vi "ExampleClient.vi"() -> ()   [LabVIEW 2013]
panel:
  out "Response":string
  out "Command":string
  in  "VarSet":T1(array[cluster])
  in  "Send Seq":bool
  in  "Send Now":bool
  in  "Send Mulligan":bool
  in  "Mulligan FileNum":i32
  in  "stop":bool
  in  "IP Address":string="127.0.0.1"
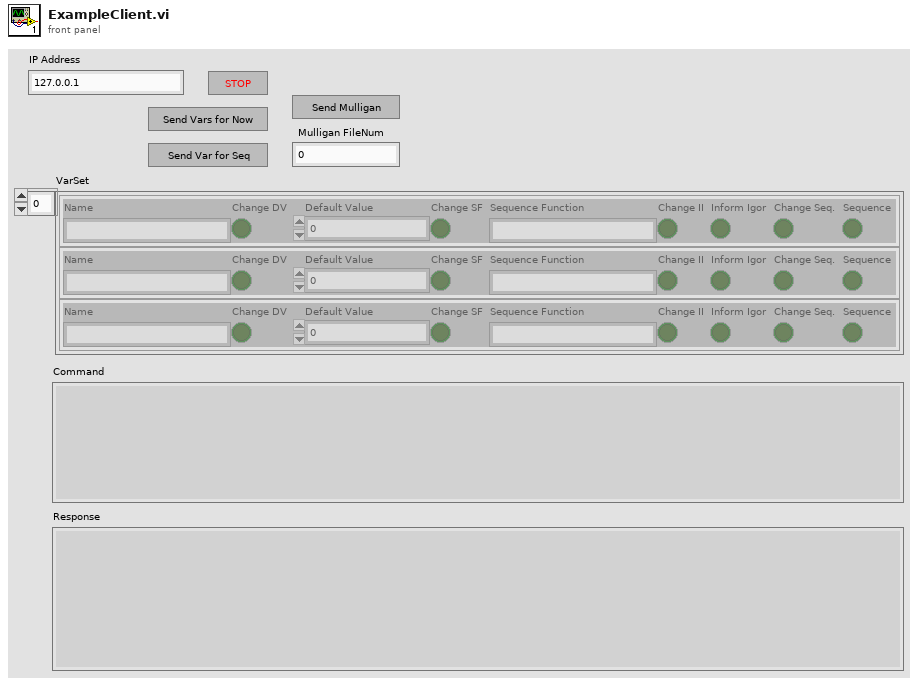
[diagram p1: front panel]
types:
  T1 = cluster{"Name":string, "Change DV":bool, "Default Value":dbl, "Change SF":bool, "Sequence Function":string, "Change II":bool, "Inform Igor":bool, "Change Seq.":bool, "Sequence":bool}[]
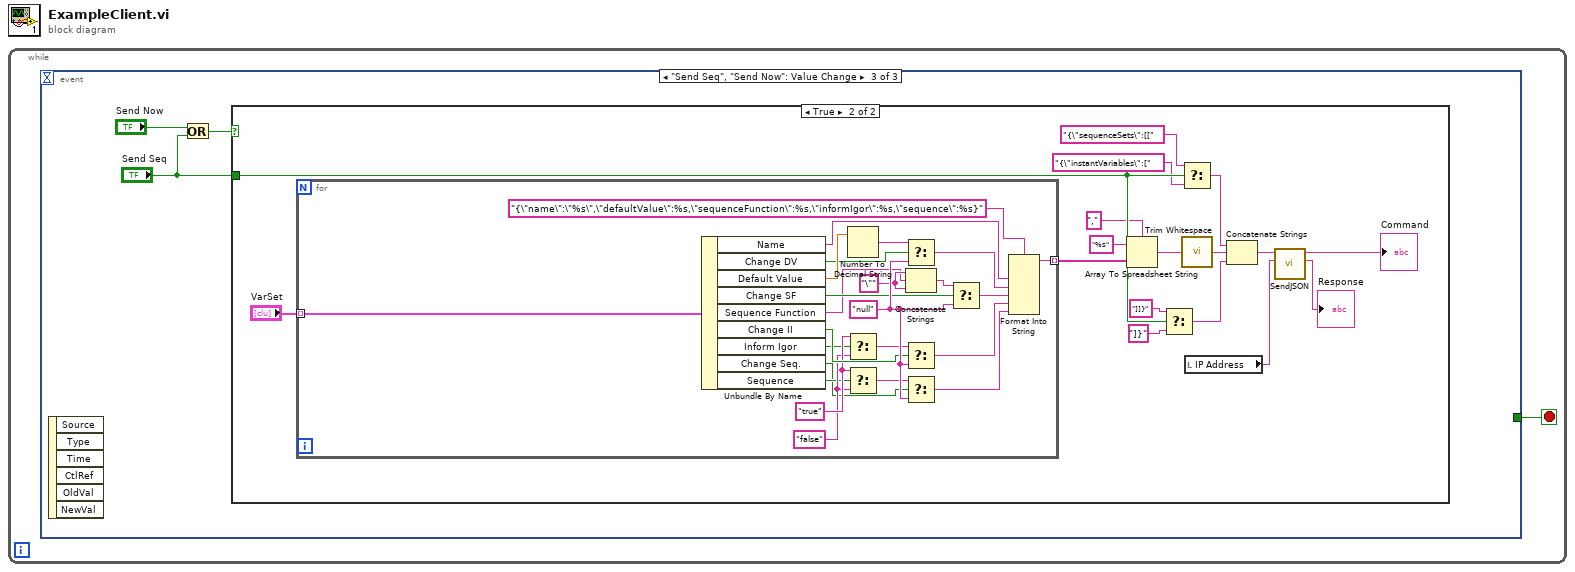
[diagram p0: block diagram]
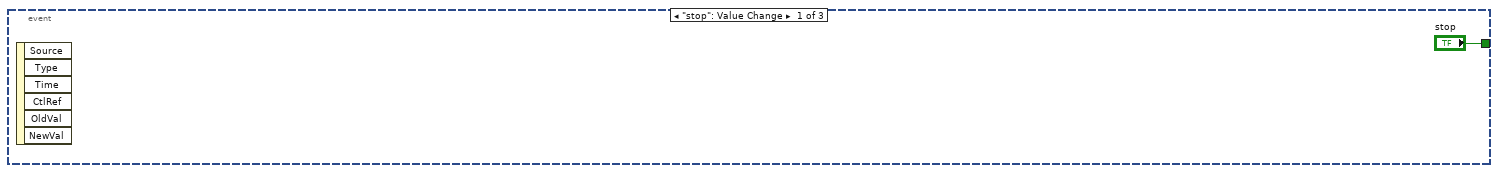
[diagram p2: hidden frame]
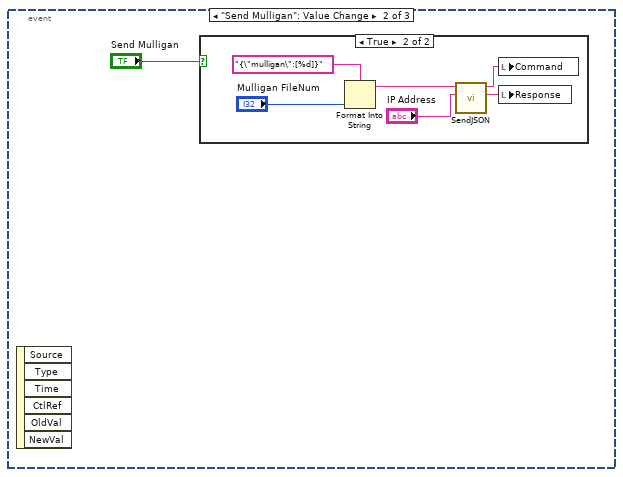
[diagram p3: hidden frame]
diagram:
  n1 = while {
    stop <- w1 stop-if-true
    n2 = event shown="[2] \"Send Seq\", \"Send Now\": Value Change" {
      selector: _ -> [_ _ _]
      dyn-events: _ -> [_ _ _]
      timeout: _ -> [_ _ _]
      tunnel: ["stop" _ _] -> w1
      event "stop": Value Change {
        n3 = event-data() -> ()  [unwired: 1 in, 6 out]
      }
      event "Send Mulligan": Value Change {
        n4 = event-data() -> ()  [unwired: 1 in, 6 out]
        n5 = case shown="True" "Send Mulligan" {
          frame False {
          }
          frame True {
            n6 = Format Into String(format string="{\"mulligan\":[%d]}" ("initial string"), "Mulligan FileNum") -> (resulting string=w5:string)  [unwired: 2 in, 1 out]
            n7 = call "SendJSON.vi"("IP Address"="IP Address", "JSON in"=w5) -> ("Response Out"=w7:string, "Command Out"=w8:string)  [unwired: 8 in]
            n8 = local write "Command"(w8) -> ()
            n9 = local write "Response"(w7) -> ()
          }
        }
      }
      event "Send Seq", "Send Now": Value Change {
        n10 = event-data() -> ()  [unwired: 1 in, 6 out]
        n11 = Or(x="Send Now", y="Send Seq") -> (x .or. y?=w11:bool)
        n12 = case shown="True" w11 {
          tunnel: "Send Seq" -> [_ w25]
          frame False {
          }
          frame True {
            n13 = for {
              tunnel: "VarSet" -> [w53] mode=indexing
              tunnel: [w39] -> w17 mode=indexing
              w32 = "\"" ("string")
              w45 = "false"
              w46 = "true"
              w49 = "null"
              n14 = Unbundle By Name(w53) -> ("Name"=w37:string, "Change DV"=w51:bool, "Default Value"=w52:dbl, "Change SF"=w48:bool, "Sequence Function"=w31:string, "Change II"=w47:bool, "Inform Igor"=w44:bool, "Change Seq."=w40:bool, "Sequence"=w43:bool)
              n15 = Number To Decimal String(number=w52) -> (decimal integer string=w50:string)  [unwired: 1 in]
              n16 = Select(t=w46, s=w44, f=w45) -> (s? t:f=w41:string)
              n17 = Select(t=w46, s=w43, f=w45) -> (s? t:f=w42:string)
              n18 = Select(t=w50, s=w51, f=w49) -> (s? t:f=w36:string)
              n19 = Concatenate Strings(w32, w31, w32) -> (w30:string)
              n20 = Select(t=w41, s=w47, f=w49) -> (s? t:f=w34:string)
              n21 = Select(t=w42, s=w40, f=w49) -> (s? t:f=w33:string)
              n22 = Select(t=w30, s=w48, f=w49) -> (s? t:f=w35:string)
              n23 = Format Into String(format string="{\"name\":\"%s\",\"defaultValue\":%s,\"sequenceFunction\":%s,\"informIgor\":%s,\"sequence\":%s}", w37, w36, w35, w34, w33) -> (resulting string=w39:string)  [unwired: 2 in, 1 out]
            }
            n24 = Array To Spreadsheet String(delimiter (Tab)=",", array=w17, 3:"%s" ("format string")) -> (spreadsheet string=w19:string)
            n25 = Select(t="]]}" ("string"), s=w25, f="]}" ("string")) -> (s? t:f=w14:string)
            n26 = Select(t="{\"sequenceSets\":[[" ("string"), s=w25, f="{\"instantVariables\":[" ("string")) -> (s? t:f=w15:string)
            n27 = call <vilib>:"Trim Whitespace.vi"("string"=w19) -> ("trimmed string"=w13:string)  [unwired: 1 in]
            n28 = local read "IP Address"() -> (w26:string)
            n29 = Concatenate Strings(w15, w13, w14) -> (w22:string)
            n30 = call "SendJSON.vi"("IP Address"=w26, "JSON in"=w22) -> ("Response Out"=→"Response":string, "Command Out"=→"Command":string)  [unwired: 8 in]
          }
        }
      }
    }
  }
